vi "Trans Coordinate.vi"(2 "CursLoc":cluster{"X":dbl, "Y":dbl}, 3 "CtlRef":refnum<vi>) -> (0 "coordinate":string, 1 "Coords":T1)   [LabVIEW 2020, in "[V] Waveform.lvlib" / "[V] Waveform.lvclass"]
uses:
  [V] Waveform.lvclass
  <vilib>/Utility/miscctls.llb/LVPoint32TypeDef.ctl
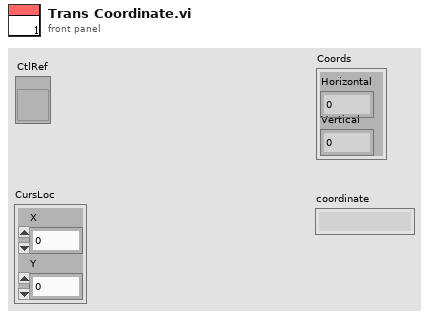
[diagram p1: front panel]
types:
  T1 = typedef "LVPoint32TypeDef.ctl" = cluster{"Horizontal":i32, "Vertical":i32}
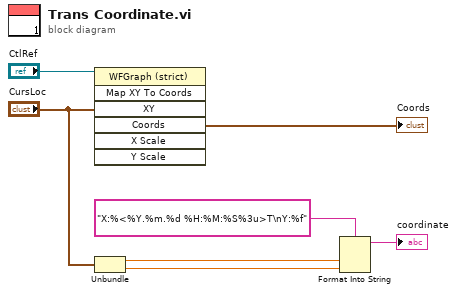
[diagram p0: block diagram]
diagram:
  n1 = invoke class="WFGraph (strict)" method="Map XY To Coords"(reference="CtlRef", "XY"="CursLoc") -> ("Coords"=→"Coords":T1)  [unwired: 5 in, 6 out]
  n2 = Unbundle("CursLoc") -> ("X"=w4:dbl, "Y"=w3:dbl)
  n3 = Format Into String(format string="X:%<%Y.%m.%d %H:%M:%S%3u>T\nY:%f", w4, w3) -> (resulting string=→"coordinate":string)  [unwired: 2 in, 1 out]
